vi "List observers.vi"(8 "error in (no error)":errorcluster, 11 "Chat in":refnum<class "Chat.lvclass">) -> (0 "error out":errorcluster, 3 "Chat out":refnum<class "Chat.lvclass">)   [LabVIEW 2012, in "Chat.lvclass"]
uses:
  Chat.lvclass
  Chat.lvclass/Chat.ctl
  person_cluster.ctl
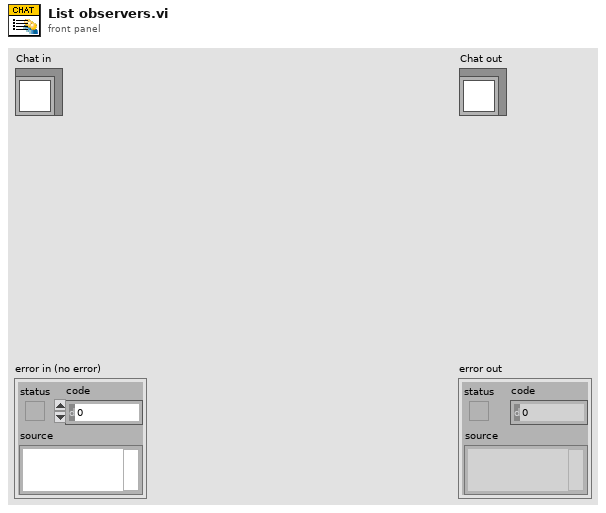
[diagram p1: front panel]
types:
  T1 = typedef "Chat.lvclass/person_cluster.ctl" = cluster{"writing?":bool, "name":string}
  T2 = typedef "Chat.lvclass/observers_cluster.ctl" = cluster{"id":string, "writing":bool}
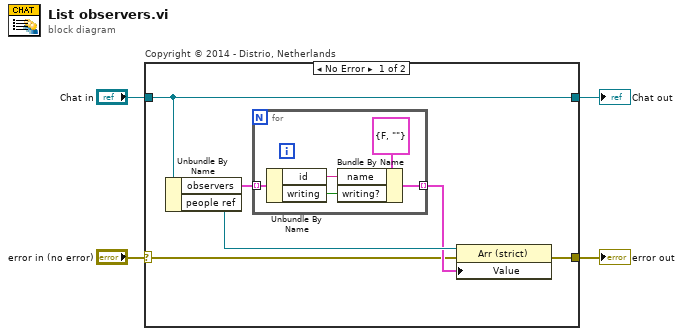
[diagram p0: block diagram]
diagram:
  n1 = case "Copyright © 2014 - Distrio, Netherlands" shown="No Error" "error in (no error)" {
    selector: "error in (no error)" -> [w5 w17]
    tunnel: [w8 w17] -> w3
    tunnel: [w6 w16] -> w1
    tunnel: "Chat in" -> [w6 w16]
    frame No Error {
      n2 = Unbundle By Name(w6) -> ("observers"=w10:T2[], "people ref"=w9:refnum<vi>)
      n3 = for {
        tunnel: [w11] -> w7 mode=indexing
        tunnel: w10 -> [w15] mode=indexing
        n4 = Unbundle By Name(w15) -> ("id"=w13:string, "writing"=w12:bool)
        n5 = Bundle By Name(cluster=T1 {"writing?"=FALSE, "name"=""} ("persons"), "name"=w13, "writing?"=w12) -> (w11:T1)
      }
      n6 = property class="Arr (strict)"(reference=w9, error in=w5, "Value"=w7) -> (error out=w8:errorcluster)  [unwired: 1 out]
    }
    frame Error {
    }
  }
  "error out" <- w3
  "Chat out" <- w1
